vi "NI_myRIO_1900_FPGA_camera_trigger.vi"() -> ()   [LabVIEW 2019]
doc: "The myRIO v1.1 FPGA Shipping Personality. This personality contains support for:\n- 2 Analog Input Interrupt channel\n- 4 Digital Input Interrupt channel\n- 1 Timer\n- 1 Accelerometer\n- 1 Button\n- 4 LED\n- 10 Analog Input channels with 1 Sample\n- 6 Analog Output channels with 1 Sample\n- 40 Digital I/O channels with 1 Sample\n- 2 I2C channels\n- 4 Encoder channels\n- 6 PWM channels\n- 2 SPI channels"
uses:
  <vilib>/rvi/Emulation/niFpgaGetClockAttributes.vi
  <vilib>/rvi/Emulation/niFpgaSctlEmulationGetInTimedLoop.vi
  <vilib>/rvi/Emulation/niFpgaEmulationReportErrorSimple.vi
  <vilib>/rvi/Emulation/niFpgaProcessEmulError.vi
  <vilib>/rvi/Emulation/niFpgaCriticalErrorInLSC.vi
  <vilib>/rvi/eio/common/nirviEmuTemplateMethod_errors.vi
  <vilib>/eio/EIONode/EIONode.xnode
panel:
  in  "Sequence":bool
  in  "SequenceSize":u64
  in  "PinArray":u8[](array[numeric])=[0, 0, 0, 0, 0, 0, 0, 0]
  out "LoopNumber":u64
  in  "OutputPinMap":u8
  out "PinMap":bool[](array[boolean])
  out "DIO_indicator":bool[](array[boolean])
  out "Camera_triggerin":bool
  out "Camera_triggerout":bool
  in  "Synchronization":bool
  in  "PulseNumberperLoop":i32
  in  "Trigger":u64
  in  "BreakinLoop":bool
  in  "OFFTime":u32
  in  "ONTime":u32
  out "PulseNumber":u64
  # "Camera trigger port: A:DIO8\nCamera trigger in: C:DIO0\nLight source port: C:DIO1~7, 1~6 are Normally Open (NO), 7 is  NC."
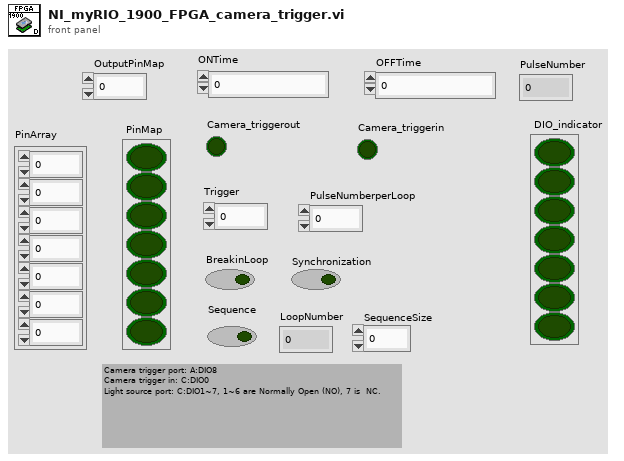
[diagram p1: front panel]
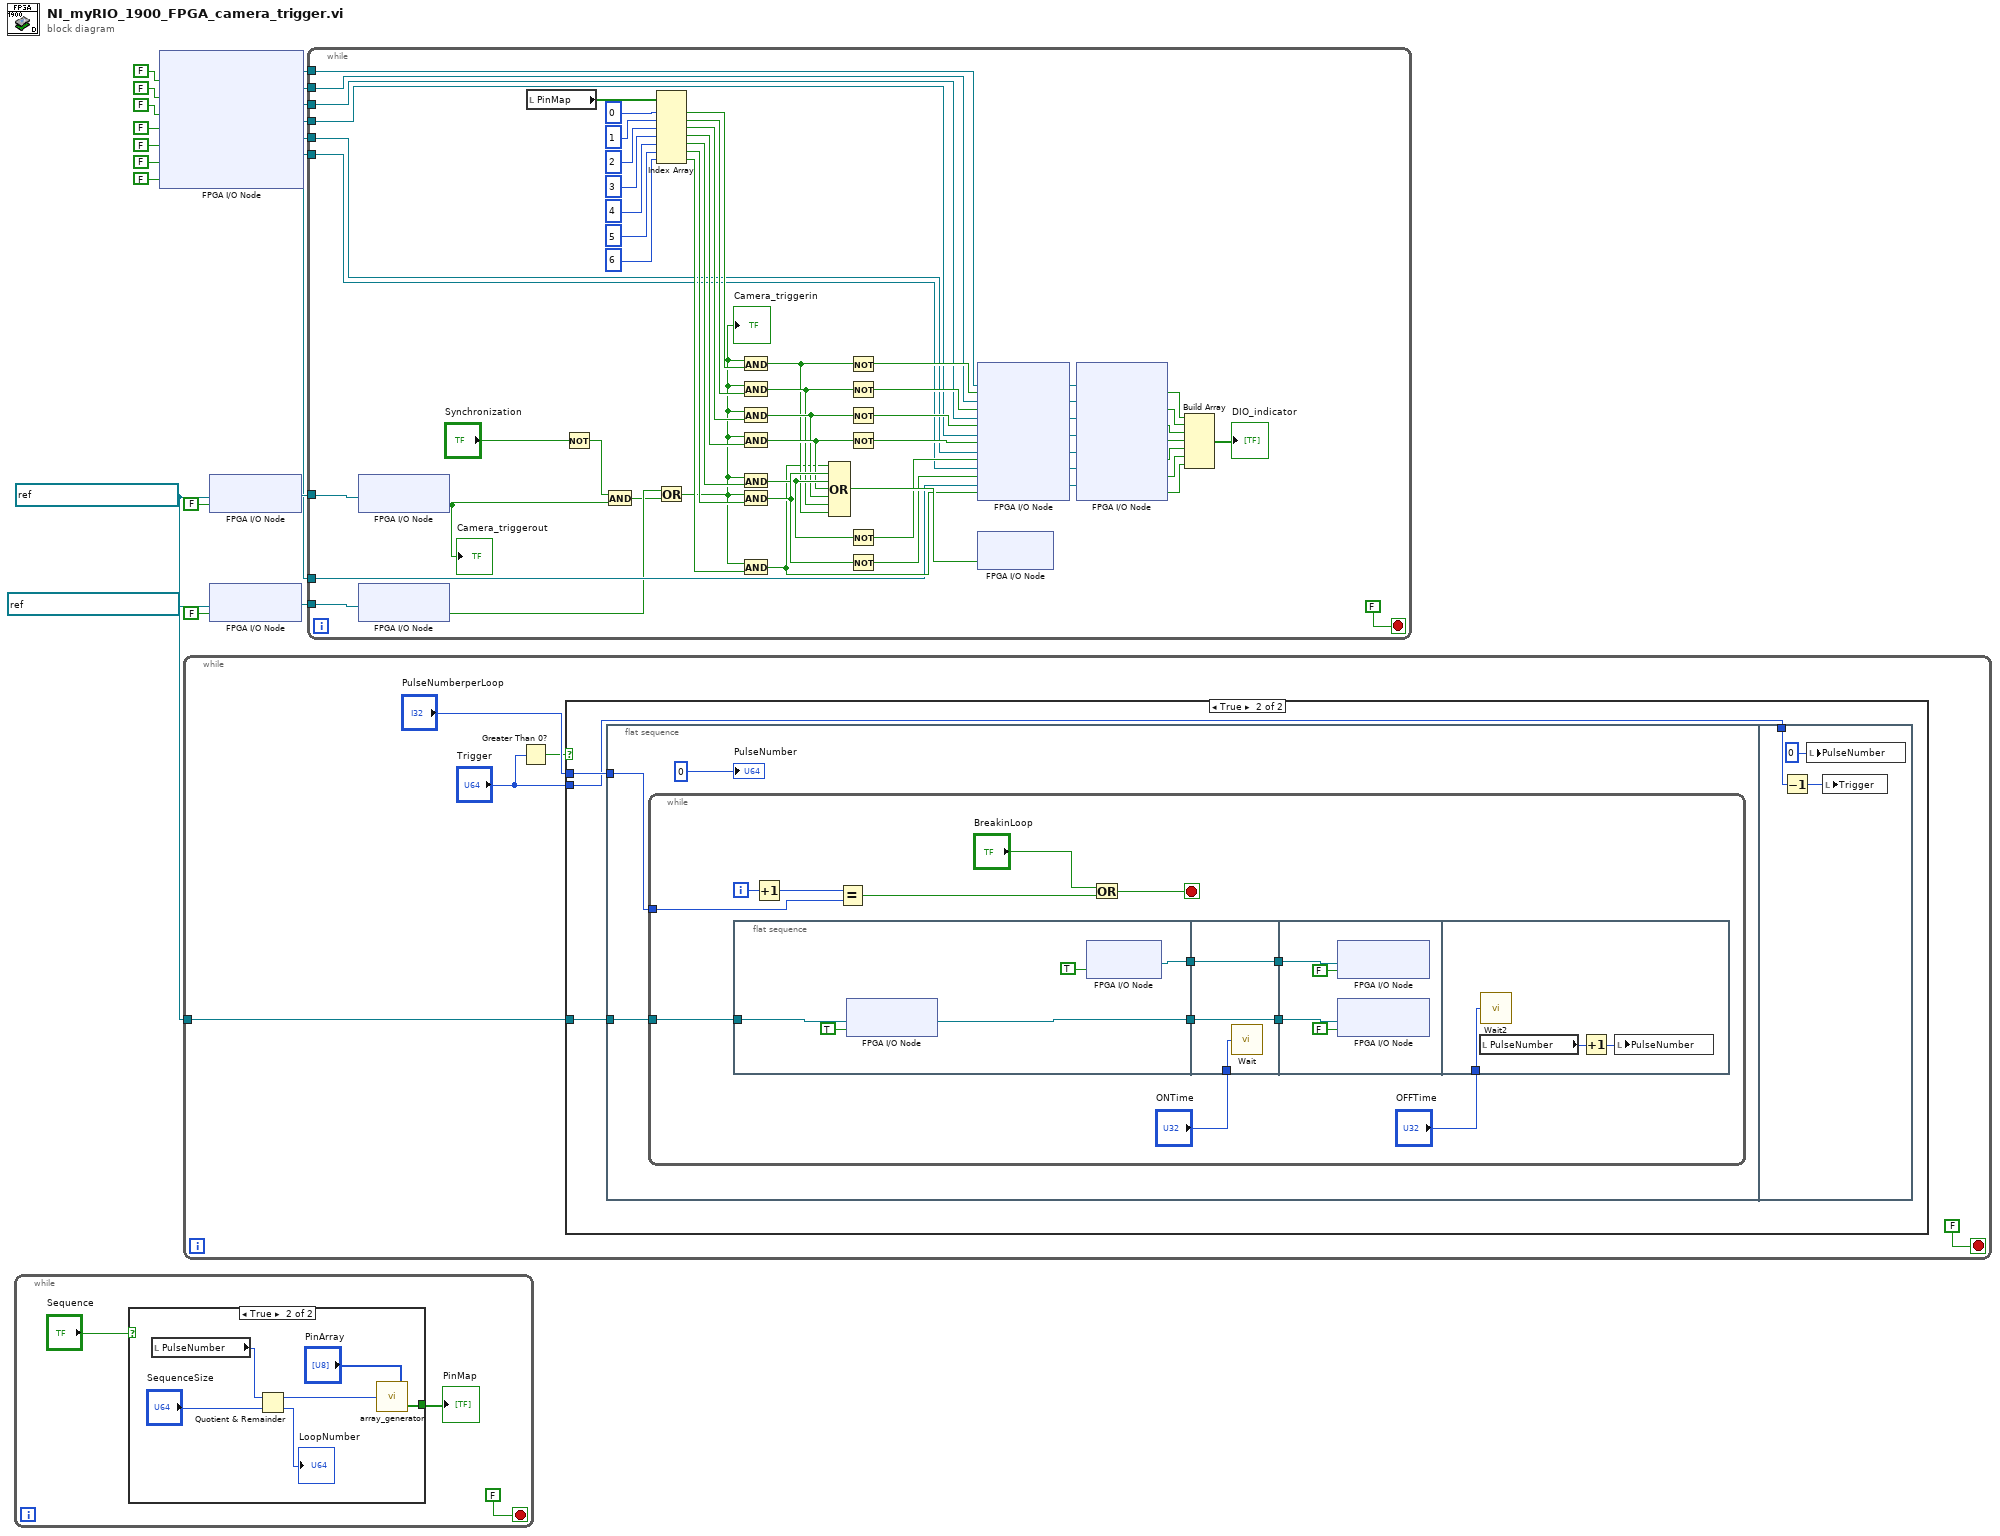
[diagram p0: block diagram]
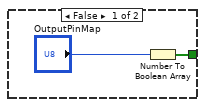
[diagram p2: hidden frame]
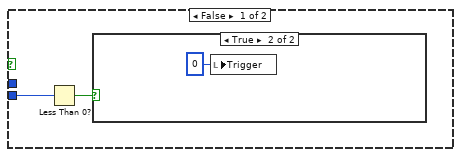
[diagram p3: hidden frame]
diagram:
  w1 = refnum<k21> "ConnectorA/DIO8" ("FPGA I/O In")
  n1 = while {
    stop <- FALSE stop-if-true
    n2 = case shown="True" "Sequence" {
      tunnel: [w24 w29] -> w22
      frame False {
        n3 = Number To Boolean Array(number="OutputPinMap") -> (Boolean array=w24:bool[])
      }
      frame True {
        n4 = local read "PulseNumber"() -> (w26:u64)
        n5 = Quotient & Remainder(x=w26, y="SequenceSize") -> (x-y*floor(x/y)=w30:u64, floor(x/y)=→"LoopNumber":u64)
        n6 = call "array_generator.vi"("Index"=w30, "Array"="PinArray") -> ("Boolean array"=w29:bool[])
      }
    }
    "PinMap" <- w22
  }
  n7 = xnode "FPGA I/O Node"("ConnectorC/DIO1"=FALSE, "ConnectorC/DIO2"=FALSE, "ConnectorC/DIO3"=FALSE, "ConnectorC/DIO4"=FALSE, "ConnectorC/DIO5"=FALSE, "ConnectorC/DIO6"=FALSE, "ConnectorC/DIO7"=FALSE) -> ("FPGA I/O Out"=w8:refnum<k21>, "FPGA I/O Out"=w7:refnum<k21>, "FPGA I/O Out"=w6:refnum<k21>, "FPGA I/O Out"=w5:refnum<k21>, "FPGA I/O Out"=w4:refnum<k21>, "FPGA I/O Out"=w3:refnum<k21>, "FPGA I/O Out"=w2:refnum<k21>)  [unwired: 7 in]
  n8 = while {
    tunnel: w1 -> [w32]
    stop <- FALSE stop-if-true
    n9 = Greater Than 0?(x="Trigger") -> (x > 0?=w35:bool)
    n10 = case shown="True" w35 {
      tunnel: "PulseNumberperLoop" -> [_ w42]
      tunnel: "Trigger" -> [w38 w41]
      tunnel: w32 -> [_ w40]
      frame False {
        n11 = Less Than 0?(x=w38) -> (x < 0?=w37:bool)
        n12 = case shown="True" w37 {
          frame False {
          }
          frame True {
            n13 = local write "Trigger"(i16 0) -> ()
          }
        }
      }
      frame True {
        n14 = flat-sequence {
          tunnel: w42 -> [w45]
          tunnel: w40 -> [w44]
          tunnel: w41 -> [w75]
          frame #0 {
            n15 = while {
              tunnel: w45 -> [w54]
              tunnel: w44 -> [w46]
              i -> [w47]
              stop <- w56 stop-if-true
              n16 = flat-sequence {
                tunnel: [w61] -> w50
                tunnel: [w60] -> w48
                tunnel: w46 -> [w59]
                tunnel: "ONTime" -> [w66]
                tunnel: [w65] -> w51
                tunnel: w50 -> [w65]
                tunnel: [w64] -> w49
                tunnel: w48 -> [w64]
                tunnel: w51 -> [w68]
                tunnel: w49 -> [w67]
                tunnel: "OFFTime" -> [w73]
                frame #0 {
                  n17 = xnode "FPGA I/O Node"("I/O Item"=TRUE ("ConnectorA/DIO8"), "FPGA I/O In"=w59) -> ("FPGA I/O Out"=w60:refnum<k21>)
                  n18 = xnode "FPGA I/O Node"("LED0"=TRUE ("ConnectorA/DIO8")) -> ("FPGA I/O Out"=w61:refnum<k21>)  [unwired: 1 in]
                }
                frame #1 {
                  n19 = call "Wait"("Count(uSec)"=w66) -> ()  [unwired: 1 out]
                }
                frame #2 {
                  n20 = xnode "FPGA I/O Node"("I/O Item"=FALSE ("ConnectorA/DIO8"), "FPGA I/O In"=w68) -> ()  [unwired: 1 out]
                  n21 = xnode "FPGA I/O Node"("I/O Item"=FALSE ("ConnectorA/DIO8"), "FPGA I/O In"=w67) -> ()  [unwired: 1 out]
                }
                frame #3 {
                  n22 = local read "PulseNumber"() -> (w72:u64)
                  n23 = call "Wait2"("Count(uSec)"=w73) -> ()  [unwired: 1 out]
                  n24 = Increment(x=w72) -> (x+1=w71:u64)
                  n25 = local write "PulseNumber"(w71) -> ()
                }
              }
              n26 = Increment(x=w47) -> (x+1=w55:i32)
              n27 = Equal?(x=w55, y=w54) -> (x = y?=w58:bool)
              n28 = Or(x="BreakinLoop", y=w58) -> (x .or. y?=w56:bool)
            }
            "PulseNumber" <- i16 0
          }
          frame #1 {
            n29 = Decrement(x=w75) -> (x-1=w76:u64)
            n30 = local write "PulseNumber"(u64 0 ("PulseNumber")) -> ()
            n31 = local write "Trigger"(w76) -> ()
          }
        }
      }
    }
  }
  n32 = xnode "FPGA I/O Node"("I/O Item"=FALSE ("ConnectorA/DIO8"), "FPGA I/O In"=w1) -> ("FPGA I/O Out"=w18:refnum<k21>)
  n33 = xnode "FPGA I/O Node"("I/O Item"=FALSE ("ConnectorB/DIO7"), "FPGA I/O In"=refnum<k21> "ConnectorA/DIO15") -> ("FPGA I/O Out"=w15:refnum<k21>)
  n34 = while {
    tunnel: w18 -> [w99]
    tunnel: w15 -> [w98]
    tunnel: w8 -> [w97]
    tunnel: w7 -> [w96]
    tunnel: w6 -> [w95]
    tunnel: w5 -> [w94]
    tunnel: w4 -> [w93]
    tunnel: w3 -> [w92]
    tunnel: w2 -> [w91]
    stop <- FALSE stop-if-true
    n35 = xnode "FPGA I/O Node"("FPGA I/O In"=w99) -> ("I/O Item"=w78:bool)  [unwired: 1 out]
    "Camera_triggerout" <- w78
    n36 = xnode "FPGA I/O Node"("FPGA I/O In"=w98) -> ("I/O Item"=w88:bool)  [unwired: 1 out]
    n37 = local read "PinMap"() -> (w77:bool[])
    n38 = Not(x="Synchronization") -> (.not. x?=w86:bool)
    n39 = And(x=w86, y=w78) -> (x .and. y?=w87:bool)
    n40 = Index Array(array=w77, index #1=0 ("index"), index #2=1 ("index"), index #3=2 ("index"), index #4=3 ("index"), index #5=4 ("index"), index #6=5 ("index"), index #7=6 ("index")) -> (element #1=w125:bool, element #2=w124:bool, element #3=w123:bool, element #4=w122:bool, element #5=w121:bool, element #6=w120:bool, element #7=w119:bool)
    n41 = Or(x=w88, y=w87) -> (x .or. y?=w89:bool)
    "Camera_triggerin" <- w89
    n42 = And(x=w89, y=w125) -> (x .and. y?=w113:bool)
    n43 = And(x=w89, y=w124) -> (x .and. y?=w114:bool)
    n44 = And(x=w89, y=w123) -> (x .and. y?=w115:bool)
    n45 = And(x=w89, y=w122) -> (x .and. y?=w116:bool)
    n46 = And(x=w89, y=w121) -> (x .and. y?=w117:bool)
    n47 = And(x=w89, y=w120) -> (x .and. y?=w118:bool)
    n48 = And(x=w89, y=w119) -> (x .and. y?=w107:bool)
    n49 = Compound Arithmetic op=OR(w107, w118, w117, w116, w115, w114, w113) -> (w112:bool)
    n50 = Not(x=w113) -> (.not. x?=w126:bool)
    n51 = Not(x=w114) -> (.not. x?=w127:bool)
    n52 = Not(x=w115) -> (.not. x?=w111:bool)
    n53 = Not(x=w116) -> (.not. x?=w110:bool)
    n54 = Not(x=w117) -> (.not. x?=w109:bool)
    n55 = Not(x=w118) -> (.not. x?=w108:bool)
    n56 = xnode "FPGA I/O Node"("I/O Item"=w126, "FPGA I/O In"=w97, "I/O Item"=w127, "FPGA I/O In"=w96, "I/O Item"=w111, "FPGA I/O In"=w95, "I/O Item"=w110, "FPGA I/O In"=w94, "I/O Item"=w109, "FPGA I/O In"=w93, "I/O Item"=w108, "FPGA I/O In"=w92, "I/O Item"=w107, "FPGA I/O In"=w91) -> ("FPGA I/O Out"=w106:refnum<k21>, "FPGA I/O Out"=w105:refnum<k21>, "FPGA I/O Out"=w104:refnum<k21>, "FPGA I/O Out"=w103:refnum<k21>, "FPGA I/O Out"=w102:refnum<k21>, "FPGA I/O Out"=w101:refnum<k21>, "FPGA I/O Out"=w100:refnum<k21>)
    n57 = xnode "FPGA I/O Node"("LED1"=w112) -> ()  [unwired: 1 in, 1 out]
    n58 = xnode "FPGA I/O Node"("FPGA I/O In"=w106, "FPGA I/O In"=w105, "FPGA I/O In"=w104, "FPGA I/O In"=w103, "FPGA I/O In"=w102, "FPGA I/O In"=w101, "FPGA I/O In"=w100) -> ("I/O Item"=w128:bool, "I/O Item"=w129:bool, "I/O Item"=w130:bool, "I/O Item"=w131:bool, "I/O Item"=w132:bool, "I/O Item"=w133:bool, "I/O Item"=w134:bool)  [unwired: 7 out]
    n59 = Build Array(w128, w129, w130, w131, w132, w133, w134) -> (→"DIO_indicator":bool[])
  }
